vi "Full CAN Init.vi"(8 "error in (no error)":errorcluster, 11 "XNET Commuication Properties":T1 {"CAN I/O Mode" items=["CAN", "CAN FD", "CAN FD + BRS"]}) -> (0 "error out":errorcluster, 1 "XNET Communication Properties Out":T1 {"CAN I/O Mode" items=["CAN", "CAN FD", "CAN FD + BRS"]})   [LabVIEW 2014, in "CAN Bus Monitor Engine.lvlib"]
uses:
  CAN Bus Monitor Engine.lvlib
  Controls/XNET Communication Properties.ctl
  Controls/CAN IO Mode.ctl
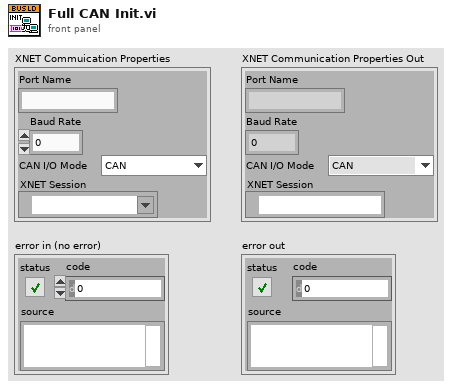
[diagram p1: front panel]
types:
  T1 = typedef "CAN Bus Monitor Engine.lvlib/XNET Communication Properties.ctl" = cluster{"Port Name":string, "Baud Rate":u32, "CAN I/O Mode":T2, "XNET Session":refnum<k21>}
  T2 = typedef "CAN Bus Monitor Engine.lvlib/CAN IO Mode.ctl" = u32
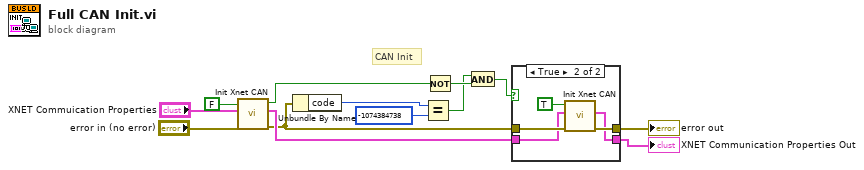
[diagram p0: block diagram]
diagram:
  # "CAN Init"
  n1 = call "Init Xnet CAN.vi"("error in"="error in (no error)", "XNET Communication Properties In"="XNET Commuication Properties", "ForceInitAsSubordinate"=FALSE) -> ("error out"=w10:errorcluster, "XNET Communication Properties Out"=w12:T1, "Init Stat"=w9:bool)  [unwired: 6 in]
  n2 = Unbundle By Name(w10) -> ("code"=w2:i32)
  n3 = Equal?(x=w2, y=-1074384738) -> (x = y?=w4:bool)
  n4 = Not(x=w9) -> (.not. x?=w6:bool)
  n5 = And(x=w4, y=w6) -> (x .and. y?=w5:bool)
  n6 = case shown="True" w5 {
    tunnel: w10 -> [w15 w19]
    tunnel: [w15 w18] -> w1
    tunnel: w12 -> [w14 w17]
    tunnel: [w14 w16] -> w13
    frame False {
    }
    frame True {
      n7 = call "Init Xnet CAN.vi"("error in"=w19, "XNET Communication Properties In"=w17, "ForceInitAsSubordinate"=TRUE) -> ("error out"=w18:errorcluster, "XNET Communication Properties Out"=w16:T1)  [unwired: 6 in, 1 out]
    }
  }
  "XNET Communication Properties Out" <- w13
  "error out" <- w1
